vi "set_custom_error.vi"(6 "name of caller in (you)":string, 8 "error in (no error)":errorcluster, 9 "custom error description":string, 10 "custom code (-1)":i32=-1) -> (0 "error out":errorcluster)   [LabVIEW 2015]
uses:
  <vilib>/Utility/error.llb/Error Code Database.vi
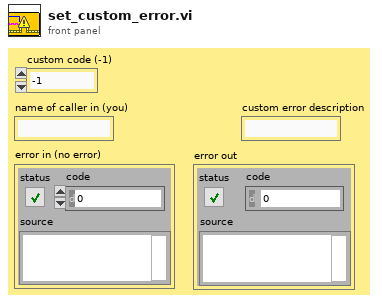
[diagram p1: front panel]
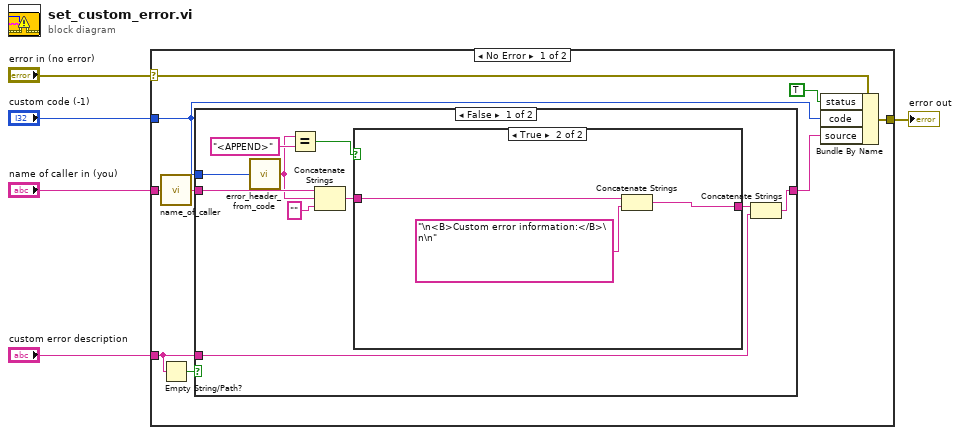
[diagram p0: block diagram]
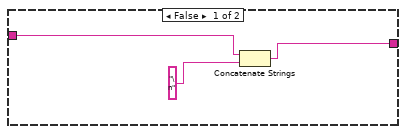
[diagram p2: hidden frame]
diagram:
  n1 = case shown="No Error" "error in (no error)" {
    selector: "error in (no error)" -> [w12 w32]
    tunnel: "name of caller in (you)" -> [w14 _]
    tunnel: "custom code (-1)" -> [w6 _]
    tunnel: [w13 w32] -> w2
    tunnel: "custom error description" -> [w9 _]
    frame No Error {
      n2 = call "name_of_caller.vi"("name of caller in"=w14) -> ("name of caller out"=w7:string)  [unwired: 3 in]
      n3 = Empty String/Path?(string/path=w9) -> (empty?=w8:bool)
      n4 = case shown="False" w8 {
        tunnel: [w21 w31] -> w10
        tunnel: w9 -> [w20 _]
        tunnel: w7 -> [w18 w31]
        tunnel: w6 -> [w16 _]
        frame False {
          n5 = call "error_header_from_code.vi"("error code"=w16) -> ("error header"=w15:string)  [unwired: 4 in]
          n6 = Equal?(x=w15, y="<APPEND>") -> (x = y?=w23:bool)
          n7 = Concatenate Strings(w18, w15, "" ("string")) -> (w17:string)
          n8 = case shown="True" w23 {
            tunnel: w17 -> [w27 w30]
            tunnel: [w26 w28] -> w22
            frame False {
              n9 = Concatenate Strings(w27, "\n" ("string")) -> (w26:string)
            }
            frame True {
              n10 = Concatenate Strings(w30, "\n<B>Custom error information:</B>\n\n" ("string")) -> (w28:string)
            }
          }
          n11 = Concatenate Strings(w22, w20) -> (w21:string)
        }
        frame True {
        }
      }
      n12 = Bundle By Name(cluster=w12, "status"=TRUE, "code"=w6, "source"=w10) -> (w13:errorcluster)
    }
    frame Error {
    }
  }
  "error out" <- w2
